vi "Find Visible Front Panels.vi"(8 "Error In":errorcluster, 10 "This VI":refnum<vi>) -> (0 "Error out":errorcluster, 2 "Running VIs":string[](array[string]))   [LabVIEW 2019, in "LSS.lvlib"]
doc: "Create list of VIs currently running on the PC that are visible.\n\n<b>Inputs:</b>\n<b>This VI</b> - The \"This VI\" reference to the calling VI. This is used such that the calling VI is excluded from the list of running VIs. Since this is used by the editor window it will edit VIs other than itself.\n<b>Error in</b> - Standard error in terminal\n\n<b>Outputs:</b>\n<b>Running VIs</b> - List of all VIs running and visible in memory.\n<b>Error out</b> - Standard error out terminal."
uses:
  LSS.lvlib
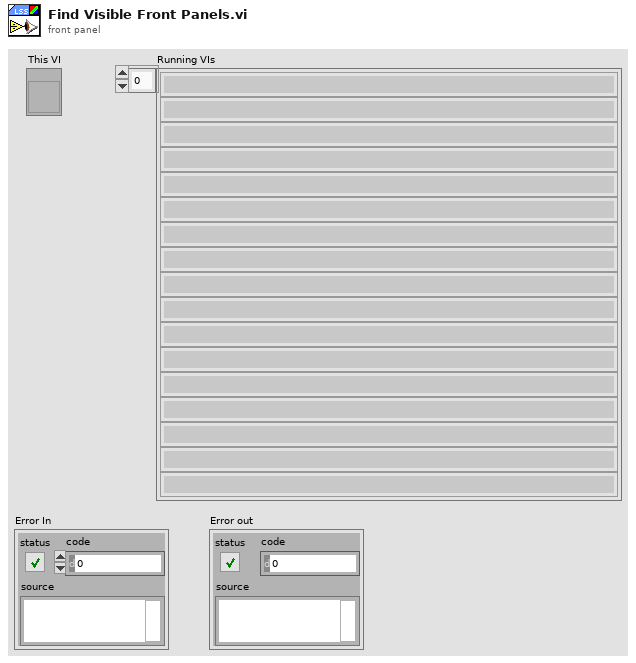
[diagram p1: front panel]
types:
  T1 = enum32{"Invalid", "Standard", "Closed", "Hidden", "Minimized", "Maximized"}
  T2 = enum32{"Bad", "Idle", "Run top level", "Running"}
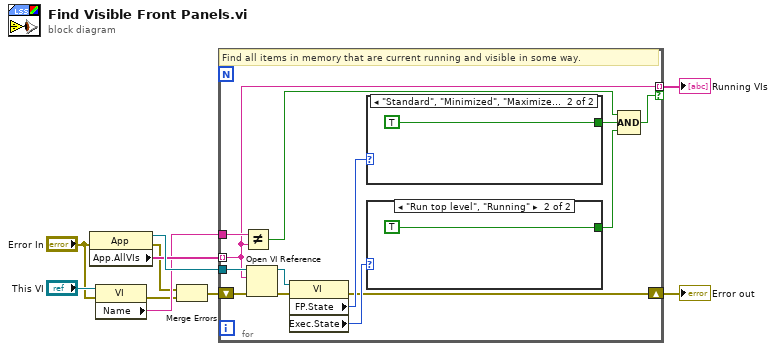
[diagram p0: block diagram]
diagram:
  n1 = property class="App"(error in="Error In") -> (reference out=w10:refnum<vi>, error out=w4:errorcluster, "App.AllVIs"=w9:string[])  [unwired: 1 in]
  n2 = property class="VI"(reference="This VI", error in="Error In") -> (error out=w1:errorcluster, "Name"=w7:string)  [unwired: 1 out]
  n3 = Merge Errors(w4, w1) -> (w2:errorcluster)
  n4 = for {
    tunnel: w10 -> [w23]
    tunnel: w9 -> [w15] mode=indexing
    tunnel: [w15] -> w8 mode=indexing if=w17
    tunnel: w7 -> [w16]
    shift-right: [w11] -> w3
    shift-left: w2 -> [w13]
    # "Find all items in memory that are current running and visible in some way."
    n5 = Not Equal?(x=w16, y=w15) -> (x != y?=w14:bool)
    n6 = Open VI Reference(application reference (local)=w23, vi path=w15, error in (no error)=w13) -> (vi reference=w22:refnum<vi>, error out=w12:errorcluster)  [unwired: 3 in]
    n7 = property class="VI"(reference=w22, error in=w12) -> (error out=w11:errorcluster, "FP.State"=w21:T1, "Exec.State"=w20:T2)  [unwired: 1 out]
    n8 = case shown="\"Standard\", \"Minimized\", \"Maximized\"" w21 {
      tunnel: [_ TRUE] -> w19
      frame "Invalid", Default {
      }
      frame "Standard", "Minimized", "Maximized" {
      }
    }
    n9 = case shown="\"Run top level\", \"Running\"" w20 {
      tunnel: [_ TRUE] -> w18
      frame "Bad", Default {
      }
      frame "Run top level", "Running" {
      }
    }
    n10 = Compound Arithmetic op=AND(w14, w19, w18) -> (w17:bool)
  }
  "Running VIs" <- w8
  "Error out" <- w3
